vi "Prepare header content.vi"(8 "error in (no error)":errorcluster, 11 "Save Image in":refnum<class "Save Image.lvclass">) -> (0 "error out":errorcluster, 2 "header_content":string, 3 "Save Image out":refnum<class "Save Image.lvclass">)   [LabVIEW 2018, in "Save Image.lvclass"]
doc: "Prepare the header content to be provided to the Python toolkit\n\nThis function returns a JSON with the information to be written into the image header"
uses:
  Save Image.lvclass
  Save Image.lvclass/Save Image.ctl
  Channel/Channel.lvclass/Channel.ctl
  Header content/Header content.lvclass/Header content.ctl
  Simulated_CCD_Camera/Simulated_CCD_Camera.lvclass
  RxTx/RxTx.lvclass
  Channel/Channel.lvclass
  Header content/Header content.lvclass
panel:
  out "ICS components":T1
  out "prev SET parameters":T2
  out "Channel information":T3
  out "CCD Config":T4
  out "Camera Status":T5
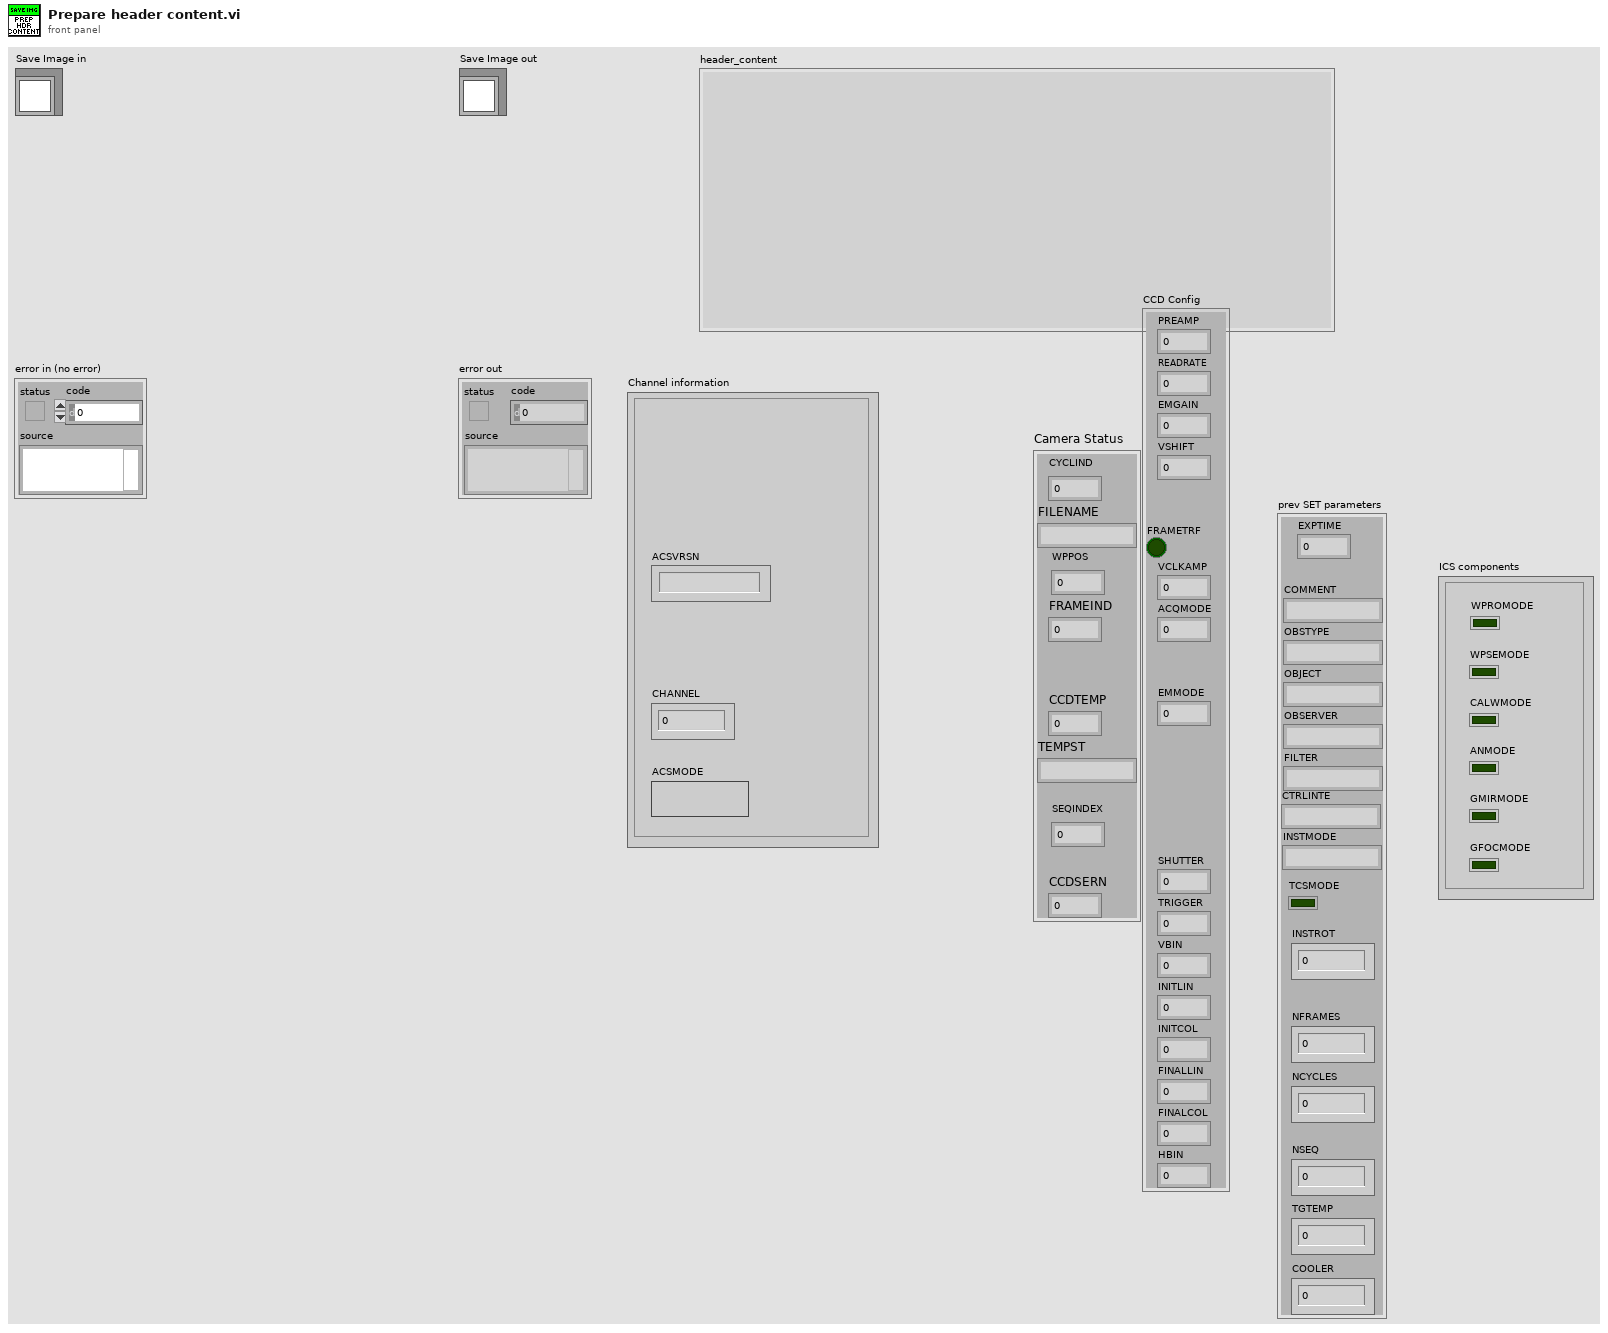
[diagram p1: front panel]
types:
  T1 = cluster{"WPSEMODE":bool, "CALWMODE":bool, "ANMODE":bool, "GMIRMODE":bool, "GFOCMODE":bool, "WPROMODE":bool}
  T2 = cluster{"EXPTIME":sgl, "COMMENT":string, "OBSTYPE":string, "OBJECT":string, "OBSERVER":string, "FILTER":string, "CTRLINTE":string, "INSTMODE":string, "TCSMODE":bool, "INSTROT":dbl, "NFRAMES":u32, "NCYCLES":u32, "NSEQ":u32, "TGTEMP":i32, "COOLER":u16}
  T3 = cluster{"ACSVRSN":string, "CHANNEL":u8, "ACSMODE":bool}
  T4 = cluster{"PREAMP":u16, "READRATE":u16, "EMGAIN":u16, "VSHIFT":u16, "FRAMETRF":bool, "VCLKAMP":u16, "ACQMODE":u16, "EMMODE":u16, "SHUTTER":u16, "TRIGGER":u16, "VBIN":u16, "INITLIN":u16, "INITCOL":u16, "FINALLIN":u16, "FINALCOL":u16, "HBIN":u16}
  T5 = cluster{"CYCLIND":u16, "FILENAME":string, "FRAMEIND":u16, "CCDTEMP":i16, "TEMPST":string, "CCDSERN":u16, "SEQINDEX":u16, "WPPOS":u8}
  T6 = cluster{"ACS mode":bool, "Image path":path, "Remote IP":string, "Python path":path, "Communication using stream":bool}
  T7 = cluster{"CYCLES_DONE":u16, "LAST_IMAGE_NAME":string, "DISK_SPACE":u16, "FRAMES_DONE":u16, "CCD_STATUS":string, "CURRENT_TEMPERATURE":i16, "TEMPERATURE_STATUS":string, "FRAME_EXPOSURE_TIME":sgl, "ERROR":bool, "SERIAL_NUMBER":u16, "ACQUIRING":bool, "IMAGE_INDEX":u32, "SEQS_DONE":u16}
  T8 = cluster{"PREAMP":u16, "READOUT_RATE":u16, "EM_GAIN":u16, "VERTICAL_SHIFT_SPEED":u16, "READ_MODE":u16, "FRAME_TRANSFER":bool, "VERTICAL_CLOCK_VOLTAGE":u16, "ACQUISITION_MODE":u16, "AD_CHANNEL":u16, "EM_MODE":u16, "SHUTTER_TTL":u16, "SHUTTER_OPENING_TIME":u16, "SHUTTER_CLOSING_TIME":u16, "SHUTTER_MODE":u16, "TRIGGER_MODE":u16, "VBIN":u16, "INITIAL_LINE":u16, "INITIAL_COLUMN":u16, "FINAL_LINE":u16, "FINAL_COLUMN":u16, "HBIN":u16}
  T9 = cluster{"COOLER_POWER_STATUS":u16, "TEMP":i32, "EXPTIME":dbl, "#FRAMES":u32, "#CYCLES":u32, "COMMENT":string, "OBSTYPE":string, "OBJECT":string, "OBSERVER":string, "FILTER":string, "CTRLINTE":string, "INSTMODE":string, "#SEQS":u32, "WAVEPLATE_POS":u16, "TCSMODE":bool, "INSTROT":dbl, "ICSMODE":u8}
  T10 = cluster{"WPROMODE":bool, "CALWMODE":bool, "ANMODE":bool, "GFOCMODE":bool, "GMIRMODE":bool, "WPSEMODE":bool}
  T11 = typedef "SYSTEMTIME structure typedef.ctl" = cluster{"Year":u16, "Month":u16, "DayOfWeek":u16, "Date":u16, "Hour":u16, "Minute":u16, "Second":u16, "Milliseconds":u16}
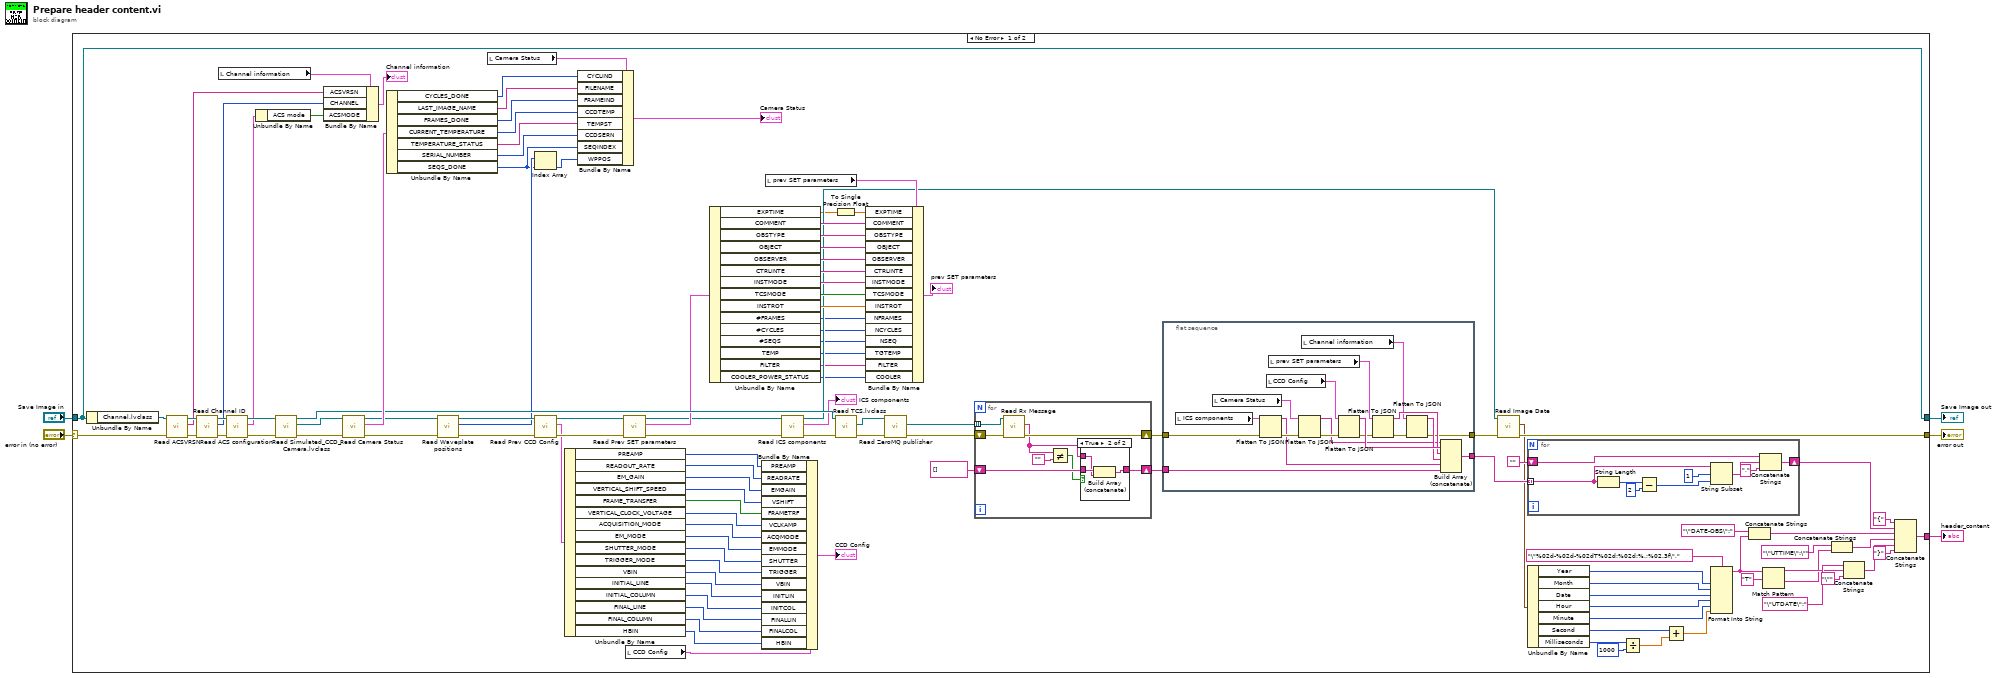
[diagram p0: block diagram]
diagram:
  n1 = case shown="No Error" "error in (no error)" {
    selector: "error in (no error)" -> [w19 w163]
    tunnel: [w102 w163] -> w4
    tunnel: [w101 w162] -> w2
    tunnel: "Save Image in" -> [w101 w162]
    tunnel: [w114 _] -> w1
    frame No Error {
      n2 = Unbundle By Name(w101) -> ("Channel.lvclass"=w23:refnum<class "Channel.lvclass">)
      n3 = call "Read ACSVRSN.vi"("error in (no error)"=w19, "Channel in"=w23) -> ("error out"=w21:errorcluster, "ACSVRSN"=w20:string, "Channel out"=w22:refnum<class "Channel.lvclass">)  [unwired: 7 in]
      n4 = call-dynamic "Read Channel ID.vi"("error in (no error)"=w21, "Channel in"=w22) -> ("error out"=w26:errorcluster, "Channel ID"=w24:u8, "Channel out"=w25:refnum<class "Channel.lvclass">)  [unwired: 7 in]
      n5 = local read "Channel information"() -> (w95:T3)
      n6 = call-dynamic "Read ACS configuration.vi"("error in (no error)"=w26, "Channel in"=w25) -> ("error out"=w53:errorcluster, "ACS configuration"=w97:T6, "Channel out"=w98:refnum<class "Channel.lvclass">)  [unwired: 7 in]
      n7 = Unbundle By Name(w97) -> ("ACS mode"=w94:bool)
      n8 = call "Read Simulated_CCD_Camera.lvclass.vi"("error in (no error)"=w53, "Channel in"=w98) -> ("error out"=w121:errorcluster, "Simulated_CCD_Camera.lvclass"=w122:refnum<class "Simulated_CCD_Camera.lvclass">, "Channel out"=w52:refnum<class "Channel.lvclass">)  [unwired: 7 in]
      n9 = Bundle By Name(cluster=w95, "ACSVRSN"=w20, "CHANNEL"=w24, "ACSMODE"=w94) -> (→"Channel information":T3)
      n10 = call "Read Camera Status.vi"("error in (no error)"=w121, "CCDCamera in"=w122) -> ("error out"=w43:errorcluster, "Camera Status"=w91:T7, "CCDCamera out"=w40:refnum<class "Simulated_CCD_Camera.lvclass">)  [unwired: 7 in]
      n11 = Unbundle By Name(w91) -> ("CYCLES_DONE"=w89:u16, "LAST_IMAGE_NAME"=w88:string, "FRAMES_DONE"=w87:u16, "CURRENT_TEMPERATURE"=w86:i16, "TEMPERATURE_STATUS"=w85:string, "SERIAL_NUMBER"=w90:u16, "SEQS_DONE"=w37:u16)
      n12 = call-dynamic "Read Waveplate positions.vi"("error in (no error)"=w43, "Simulated_CCD_Camera in"=w40) -> ("error out"=w42:errorcluster, "Waveplate positions"=w38:u8[], "Simulated_CCD_Camera out"=w41:refnum<class "Simulated_CCD_Camera.lvclass">)  [unwired: 7 in]
      n13 = local read "Camera Status"() -> (w92:T5)
      n14 = Index Array(array=w38, index=w37) -> (element=w39:u8)
      n15 = call-dynamic "Read Prev CCD Config.vi"("error in (no error)"=w42, "Simulated_CCD_Camera in"=w41) -> ("error out"=w119:errorcluster, "Prev CCD Config"=w82:T8, "Simulated_CCD_Camera out"=w120:refnum<class "Simulated_CCD_Camera.lvclass">)  [unwired: 7 in]
      n16 = Unbundle By Name(w82) -> ("PREAMP"=w81:u16, "READOUT_RATE"=w80:u16, "EM_GAIN"=w79:u16, "VERTICAL_SHIFT_SPEED"=w78:u16, "FRAME_TRANSFER"=w77:bool, "VERTICAL_CLOCK_VOLTAGE"=w76:u16, "ACQUISITION_MODE"=w75:u16, "EM_MODE"=w74:u16, "SHUTTER_MODE"=w73:u16, "TRIGGER_MODE"=w72:u16, "VBIN"=w71:u16, "INITIAL_LINE"=w70:u16, "INITIAL_COLUMN"=w69:u16, "FINAL_LINE"=w68:u16, "FINAL_COLUMN"=w67:u16, "HBIN"=w66:u16)
      n17 = Bundle By Name(cluster=w92, "CYCLIND"=w89, "FILENAME"=w88, "FRAMEIND"=w87, "CCDTEMP"=w86, "TEMPST"=w85, "CCDSERN"=w90, "SEQINDEX"=w37, "WPPOS"=w39) -> (→"Camera Status":T5)
      n18 = call-dynamic "Read Prev SET parameters.vi"("error in (no error)"=w119, "Simulated_CCD_Camera in"=w120) -> ("error out"=w32:errorcluster, "Old SET parameters"=w51:T9, "Simulated_CCD_Camera out"=w33:refnum<class "Simulated_CCD_Camera.lvclass">)  [unwired: 7 in]
      n19 = local read "CCD Config"() -> (w83:T4)
      n20 = Unbundle By Name(w51) -> ("EXPTIME"=w28:dbl, "COMMENT"=w49:string, "OBSTYPE"=w48:string, "OBJECT"=w47:string, "OBSERVER"=w46:string, "CTRLINTE"=w45:string, "INSTMODE"=w44:string, "TCSMODE"=w35:bool, "INSTROT"=w34:dbl, "#FRAMES"=w16:u32, "#CYCLES"=w17:u32, "#SEQS"=w18:u32, "TEMP"=w15:i32, "FILTER"=w14:string, "COOLER_POWER_STATUS"=w6:u16)
      n21 = Bundle By Name(cluster=w83, "PREAMP"=w81, "READRATE"=w80, "EMGAIN"=w79, "VSHIFT"=w78, "FRAMETRF"=w77, "VCLKAMP"=w76, "ACQMODE"=w75, "EMMODE"=w74, "SHUTTER"=w73, "TRIGGER"=w72, "VBIN"=w71, "INITLIN"=w70, "INITCOL"=w69, "FINALLIN"=w68, "FINALCOL"=w67, "HBIN"=w66) -> (→"CCD Config":T4)
      n22 = local read "prev SET parameters"() -> (w50:T2)
      n23 = call-dynamic "Read ICS components.vi"("error in (no error)"=w32, "Simulated_CCD_Camera in"=w33) -> ("error out"=w31:errorcluster, "ICS components"=→"ICS components":T10, "Simulated_CCD_Camera out"=w30:refnum<class "Simulated_CCD_Camera.lvclass">)  [unwired: 7 in]
      n24 = To Single Precision Float(number=w28) -> (single precision float=w27:sgl)
      n25 = call-dynamic "Read TCS.lvclass.vi"("error in (no error)"=w31, "Channel in"=w52) -> ("error out"=w12:errorcluster, "TCS.lvclass"=w13:refnum<class "Header content.lvclass">)  [unwired: 7 in, 1 out]
      n26 = Bundle By Name(cluster=w50, "EXPTIME"=w27, "COMMENT"=w49, "OBSTYPE"=w48, "OBJECT"=w47, "OBSERVER"=w46, "CTRLINTE"=w45, "INSTMODE"=w44, "TCSMODE"=w35, "INSTROT"=w34, "NFRAMES"=w16, "NCYCLES"=w17, "NSEQ"=w18, "TGTEMP"=w15, "FILTER"=w14, "COOLER"=w6) -> (→"prev SET parameters":T2)
      n27 = call "Read ZeroMQ publisher.vi"("error in (no error)"=w12, "Header content in"=w13) -> ("error out"=w11:errorcluster, "ZeroMQ publisher"=w10:refnum<class "RxTx.lvclass">[])  [unwired: 7 in, 1 out]
      n28 = for {
        tunnel: w10 -> [w130] mode=indexing
        shift-right: [w128] -> w9
        shift-left: w11 -> [w129]
        shift-right: [w127] -> w8
        shift-left: string[] [] -> [w126]
        n29 = call "Read Rx Message.vi"("error in (no error)"=w129, "RxTx in"=w130) -> ("error out"=w128:errorcluster, "Rx Message"=w125:string)  [unwired: 7 in, 1 out]
        n30 = Not Equal?(x=w125, y="") -> (x != y?=w123:bool)
        n31 = case shown="True" w123 {
          tunnel: [w131 w134] -> w127
          tunnel: w126 -> [w131 w133]
          tunnel: w125 -> [_ w132]
          frame False {
          }
          frame True {
            n32 = Build Array (concatenate)(w133, w132) -> (w134:string[])
          }
        }
      }
      n33 = flat-sequence {
        tunnel: [w151] -> w103
        tunnel: [w155] -> w115
        tunnel: w9 -> [w145]
        tunnel: w8 -> [w144]
        frame #0 {
          n34 = local read "ICS components"() -> (w148:T1)
          n35 = local read "Camera Status"() -> (w161:T5)
          n36 = Flatten To JSON(anything=w148, error in (no error)=w145) -> (JSON string=w146:string, 11:w147:errorcluster)  [unwired: 1 in]
          n37 = local read "CCD Config"() -> (w160:T4)
          n38 = local read "prev SET parameters"() -> (w150:T2)
          n39 = Flatten To JSON(anything=w161, error in (no error)=w147) -> (JSON string=w149:string, 11:w157:errorcluster)  [unwired: 1 in]
          n40 = local read "Channel information"() -> (w152:T3)
          n41 = Flatten To JSON(anything=w160, error in (no error)=w157) -> (JSON string=w159:string, 11:w156:errorcluster)  [unwired: 1 in]
          n42 = Flatten To JSON(anything=w150, error in (no error)=w156) -> (JSON string=w158:string, 11:w154:errorcluster)  [unwired: 1 in]
          n43 = Flatten To JSON(anything=w152, error in (no error)=w154) -> (JSON string=w153:string, 11:w151:errorcluster)  [unwired: 1 in]
          n44 = Build Array (concatenate)(w149, w159, w158, w153, w146, w144) -> (w155:string[])
        }
      }
      n45 = call-dynamic "Read Image Date.vi"("error in (no error)"=w103, "Simulated_CCD_Camera in"=w30) -> ("error out"=w102:errorcluster, "SYSTEMTIME"=w100:T11)  [unwired: 7 in, 1 out]
      n46 = for {
        tunnel: w115 -> [w142] mode=indexing
        shift-right: [w141] -> w99
        shift-left: "" -> [w138]
        n47 = String Length(string=w142) -> (length=w137:i32)
        n48 = Subtract(x=w137, y=2) -> (x-y=w136:i32)
        n49 = String Subset(string=w142, offset (0)=1, length (rest)=w136) -> (substring=w140:string)
        n50 = Concatenate Strings(w138, w140, ",") -> (w141:string)
      }
      n51 = Unbundle By Name(w100) -> ("Year"=w113:u16, "Month"=w112:u16, "Date"=w111:u16, "Hour"=w110:u16, "Minute"=w109:u16, "Second"=w106:u16, "Milliseconds"=w108:u16)
      n52 = Divide(x=w108, y=1000) -> (x/y=w107:dbl)
      n53 = Add(x=w106, y=w107) -> (x+y=w105:dbl)
      n54 = Format Into String(format string="\"%02d-%02d-%02dT%02d:%02d:%.;%02.3f\",", w113, w112, w111, w110, w109, w105) -> (resulting string=w65:string)  [unwired: 2 in, 1 out]
      n55 = Concatenate Strings("\"DATE-OBS\":" ("format string"), w65) -> (w63:string)
      n56 = Match Pattern(string=w65, regular expression="T") -> (before substring=w61:string, after substring=w56:string)  [unwired: 1 in, 2 out]
      n57 = Concatenate Strings("\"UTTIME\":\"" ("format string"), w56) -> (w55:string)
      n58 = Concatenate Strings("\"UTDATE\":" ("format string"), w61, "\"") -> (w54:string)
      n59 = Concatenate Strings("{", w99, w63, w55, w54, "}") -> (w114:string)
    }
    frame Error {
    }
  }
  "error out" <- w4
  "Save Image out" <- w2
  "header_content" <- w1
